vi "_csm_System_Language.vi"() -> (3 "LangID":string)   [LabVIEW 2017]
uses:
  Communicable State Machine.lvlib
  _Shared/CSM Shared.lvlib
panel:
  out "standard output":string
  out "Array of Strings":string[](array[string])
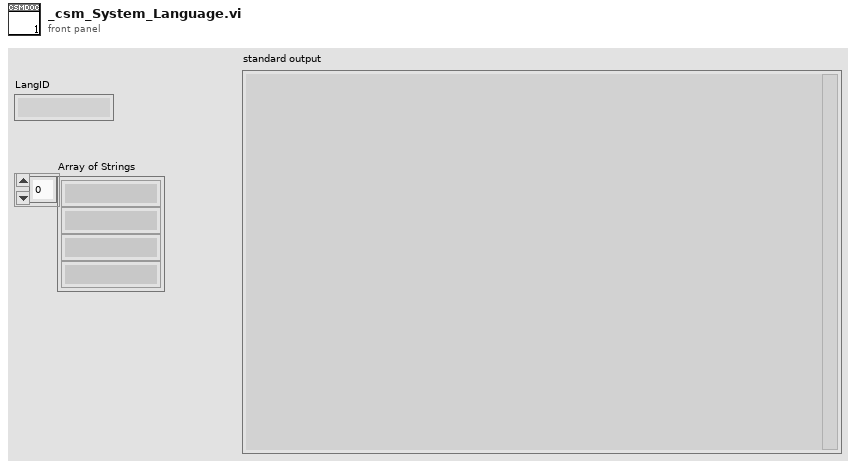
[diagram p1: front panel]
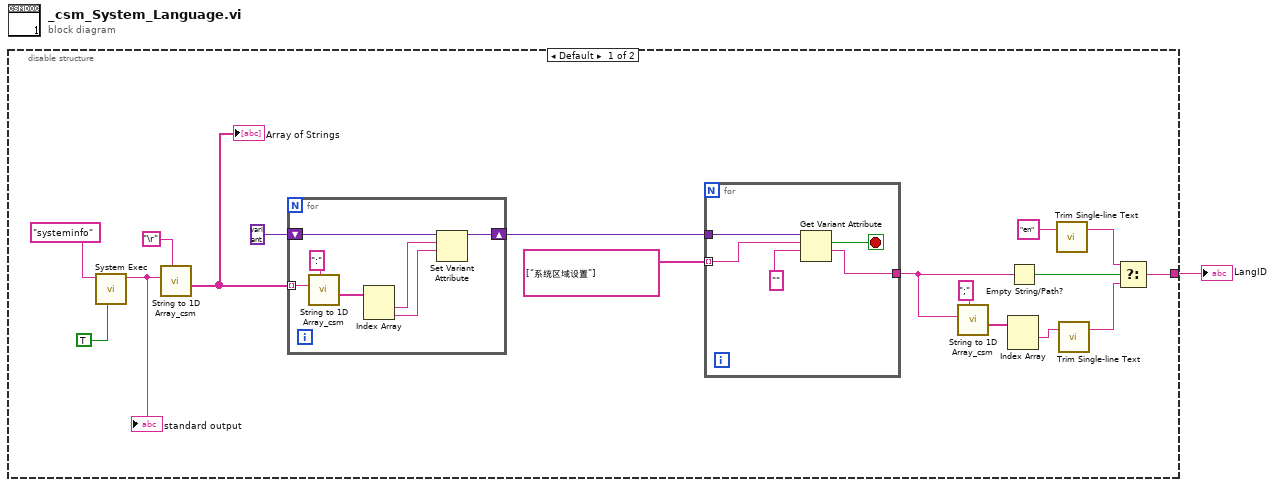
[diagram p0: block diagram]
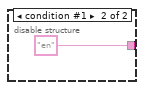
[diagram p2: hidden frame]
diagram:
  n1 = disable-structure shown="Default" {
    disable-tunnel: [w9 "en" ("trimmed string")] -> w1
    frame condition #0 (active) {
      n2 = call <vilib>:"System Exec.vi"("run minimized? (F)"=TRUE, "command line"="systeminfo") -> ("standard output"=w16:string)  [unwired: 6 in, 3 out]
      "standard output" <- w16
      n3 = call "String to 1D Array_csm.vi"("delimiter (Tab)"="\r", "string"=w16) -> ("Array of Strings"=w14:string[])  [unwired: 9 in]
      "Array of Strings" <- w14
      n4 = for {
        tunnel: w14 -> [w30] mode=indexing
        shift-right: [w27] -> w12
        shift-left: variant -> [w28]
        n5 = call "String to 1D Array_csm.vi"("delimiter (Tab)"=":", "string"=w30) -> ("Array of Strings"=w26:string[])  [unwired: 9 in]
        n6 = Index Array(array=w26) -> (element #1=w25:string, element #2=w24:string)  [unwired: 2 in]
        n7 = Set Variant Attribute(Variant=w28, name=w25, value=w24) -> (Variant out=w27:variant)  [unwired: 1 in, 2 out]
      }
      n8 = for {
        tunnel: w12 -> [w23]
        tunnel: string[] ["系统区域设置"] ("name") -> [w22] mode=indexing
        tunnel: [w19] -> w6
        stop <- w21 stop-if-true
        n9 = Get Variant Attribute(Variant=w23, name=w22, default value (empty Variant)="" ("name")) -> (found=w21:bool, value=w19:string)  [unwired: 1 in, 2 out]
      }
      n10 = call "String to 1D Array_csm.vi"("delimiter (Tab)"=";", "string"=w6) -> ("Array of Strings"=w5:string[])  [unwired: 9 in]
      n11 = Index Array(array=w5) -> (element #1=w4:string)  [unwired: 2 in, 1 out]
      n12 = Empty String/Path?(string/path=w6) -> (empty?=w10:bool)
      n13 = call "Trim Single-line Text.vi"("single-line text"="en" ("f")) -> ("trimed text"=w3:string)  [unwired: 2 in]
      n14 = call "Trim Single-line Text.vi"("single-line text"=w4) -> ("trimed text"=w2:string)  [unwired: 2 in]
      n15 = Select(t=w3, s=w10, f=w2) -> (s? t:f=w9:string)
    }
    frame condition #1 {
    }
  }
  "LangID" <- w1
